vi "Set VI Server Logging.vi"   [LabVIEW 2026]
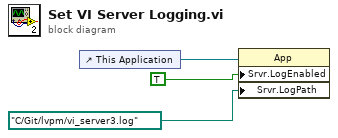
[diagram p0: block diagram]
diagram:
  n1 = control-ref of="This Application"() -> (w3:refnum<vi>)
  n2 = property class="App"(reference=w3, "Srvr.LogEnabled"=TRUE ("Server:Logging Enabled"), "Srvr.LogPath"=path "C:/Git/lvpm/vi_server3.log" ("Server:Logging File Path")) -> ()  [unwired: 1 in, 2 out]
